vi "L1RightToCargo8.vi"(9 "Initialized":bool) -> (2 "Drive State":T1)   [LabVIEW 2018]
uses:
  driveStateEnum.ctl
  L1RightToCargo8.ctl
  driveShifterEnum.ctl
  HatchPanel/hatchPanelEnum.ctl
  HatchPanel/hatchPanelNotifierCluster.ctl
  MotionProfile/Constants.vi
panel:
  out "Speed (ft/s) 3":dbl=5.820510365604576
  in  "Wait til slower then(ft/s) 3":dbl=-3.0
  out "Speed (ft/s) 2":dbl=5.820510365604576
  in  "Wait til slower then(ft/s) 2":dbl=-3.0
  out "Speed (ft/s)":dbl=5.820510365604576
  in  "Wait til slower then(ft/s)":dbl=-3.0
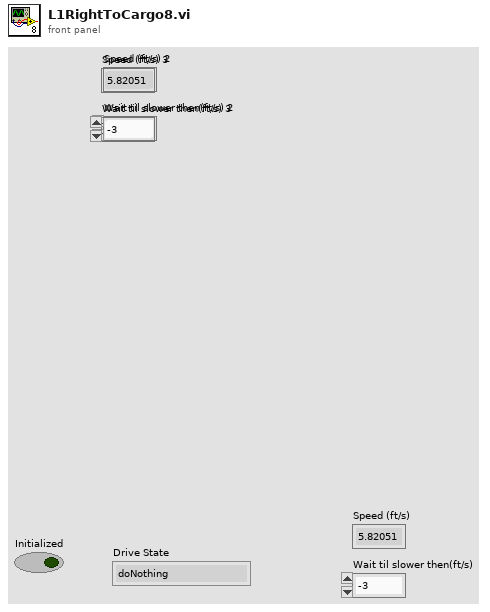
[diagram p1: front panel]
types:
  T1 = typedef "driveStateEnum.ctl" = enum16{"doNothing", "Manuel", "Teleop", "Follow Path (init)", "Follow Path", "Move to Target", "Climb", "Line Align", "Rotate180", "Align50Degrees", "Sonar Brake Tele", "LLCushion", "Auto Approach Target"}
  T2 = typedef "L1RightToCargo8.ctl" = enum16{"7b -  back away from cargo ship ", "1 - MP move to cargo Ship (init)", "2 - MP move to cargo ship", "3 - Delay for shift", "4 - Approach To Score", "5 - Scored", "99 - doNothing", "7a - back away from cargo ship (init)", "8 - Hatch Panel Motion Off", "9 - Scoring Claw On", "8 - turn towards loading station", "10 - Scoring Claw Off", "11 - MP move towards loading station (init)", "12 -  MP move towards loading station", "13 - MP Move towards  cargo ship *2 (init)", "14 - MP Move towards  cargo ship *2"}
  T3 = typedef "WPI_MotorControlDeviceRef.ctl" = cluster{"DeviceStatus":errorcluster, "Type":T4, "PWM":cluster{"PWM Channel":T5, "DeadBand":T6}, "CAN":cluster{"Device Number":u8, "SetOutput VI Ref":variant, "GetOutput VI Ref":variant, "Enable VI Ref":variant, "Disable VI Ref":variant, "Data":variant}, "Invert":bool, "DIO PWM":cluster{"PWM \"Enable\" Channel":T5, "DIOChannel":T7, "PWM Rate":dbl}}
  T4 = typedef "WPI_MotorControlType.ctl" = enum16{"PWM", "CAN", "DIO PWM"}
  T5 = typedef "FPGA_DIOPWMChannel.ctl" = enum8{"PWM 0", "PWM 1", "PWM 2", "PWM 3", "PWM 4", "PWM 5", "PWM 6", "PWM 7", "PWM 8", "PWM 9", "PWM MXP 0", "PWM MXP 1", "PWM MXP 2", "PWM MXP 3", "PWM MXP 4", "PWM MXP 5", "PWM MXP 6", "PWM MXP 7", "PWM MXP 8", "PWM MXP 9", "Invalid"}
  T6 = typedef "WPI_PWMDeadband.ctl" = cluster{"Name":string, "maxPositivePwm":i32, "minPositivePwm":i32, "centerPwm":i32, "maxNegativePwm":i32, "minNegativePwm":i32, "angularRange":u16}
  T7 = typedef "FPGA_DIOChannel.ctl" = enum8{"DIO 0", "DIO 1", "DIO 2", "DIO 3", "DIO 4", "DIO 5", "DIO 6", "DIO 7", "DIO 8", "DIO 9", "DIO MXP 0", "DIO MXP 1", "DIO MXP 2", "DIO MXP 3", "DIO MXP 4", "DIO MXP 5", "DIO MXP 6", "DIO MXP 7", "DIO MXP 8", "DIO MXP 9", "DIO MXP 10", "DIO MXP 11", "DIO MXP 12", "DIO MXP 13", "DIO MXP 14", "DIO MXP 15", "SPI Port CS1", "SPI Port CS2", "SPI Port CS3", "SPI Port MISO", "SPI Port MOSI", "Invalid"}
  T8 = typedef "driveShifterEnum.ctl" = enum16{"Low", "High"}
  T9 = typedef "hatchPanelNotifierCluster.ctl" = cluster{"Hatch Panel State":T10, "Mechanism Motion":bool, "Gathering Claw Motion":bool, "Scoring Claw Motion":bool}
  T10 = typedef "hatchPanelEnum.ctl" = enum16{"do nothing", "State Machine", "Stach Mode", "Climb Mode", "Retracted Closed", "Retracted Open", "Extended Closed", "Extended Open"}
  T11 = typedef "CTRE_PigeonIMU_DeviceRef.ctl" = cluster{"DeviceStatus":errorcluster, "Device Number":u8, "Type":T12, "Device ID":u32, "Handle":u64, "UsageFrame":u32, "Library Path":path}
  T12 = typedef "CTRE_PigeonIMU_ConnectionType.ctl" = u32
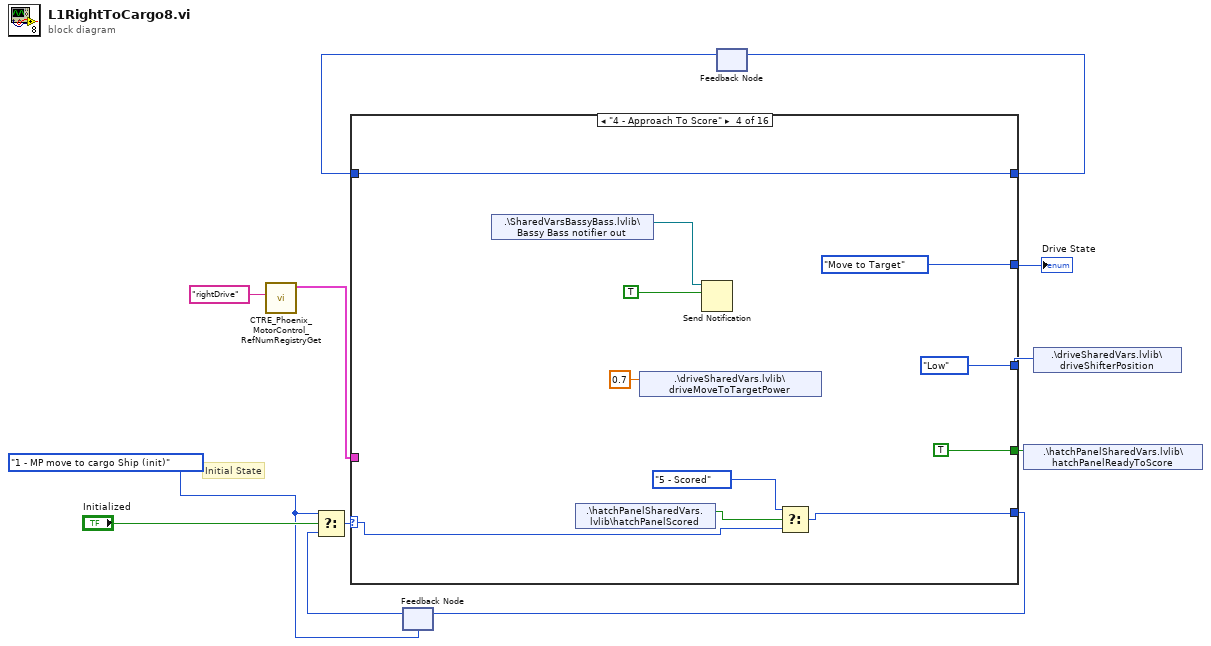
[diagram p0: block diagram]
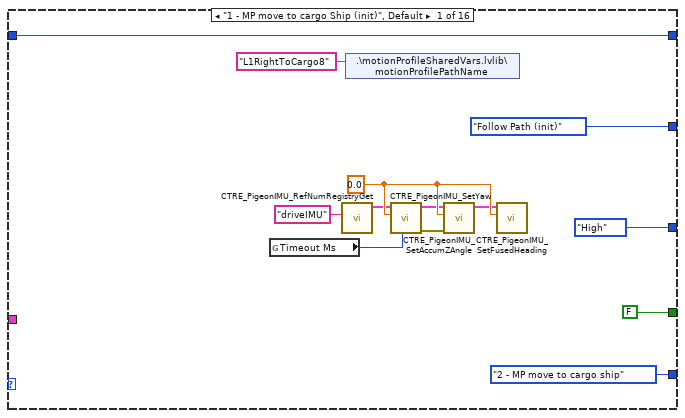
[diagram p2: hidden frame]
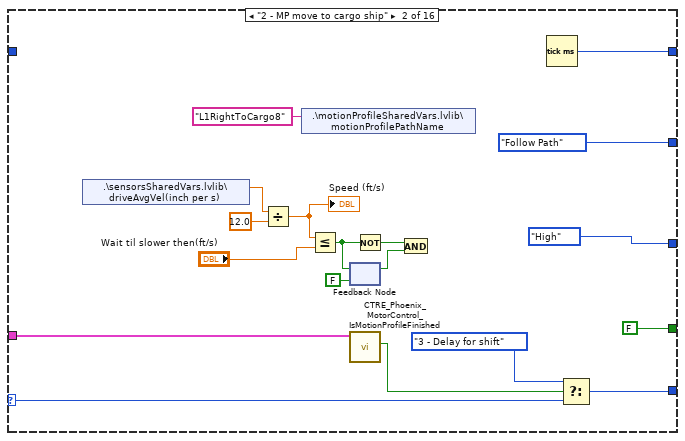
[diagram p3: hidden frame]
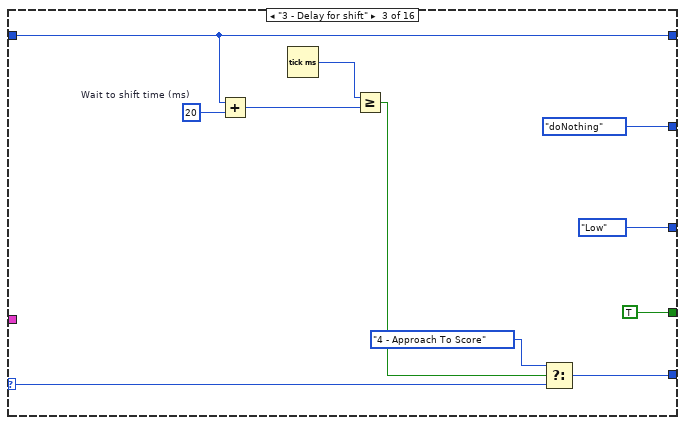
[diagram p4: hidden frame]
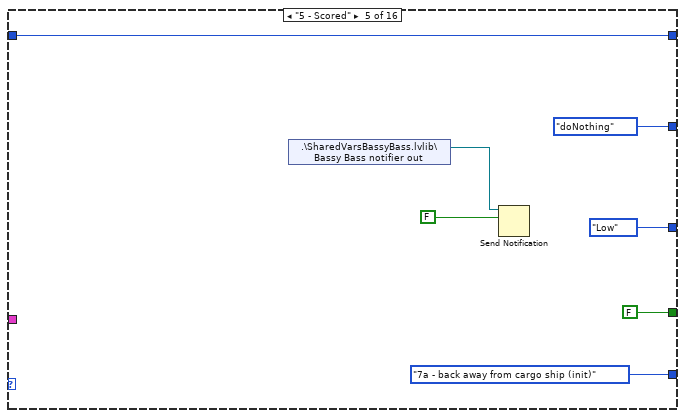
[diagram p5: hidden frame]
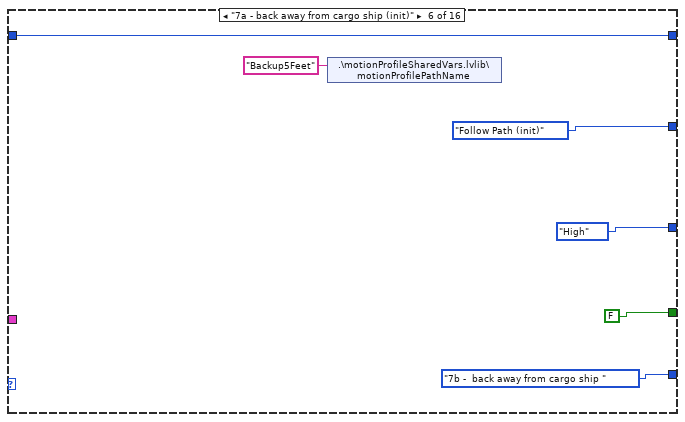
[diagram p6: hidden frame]
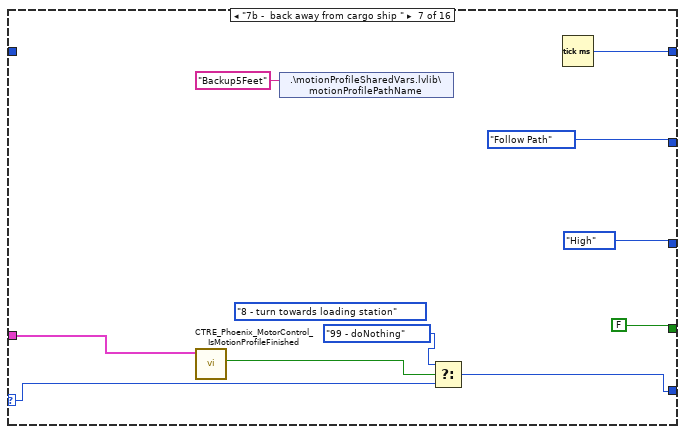
[diagram p7: hidden frame]
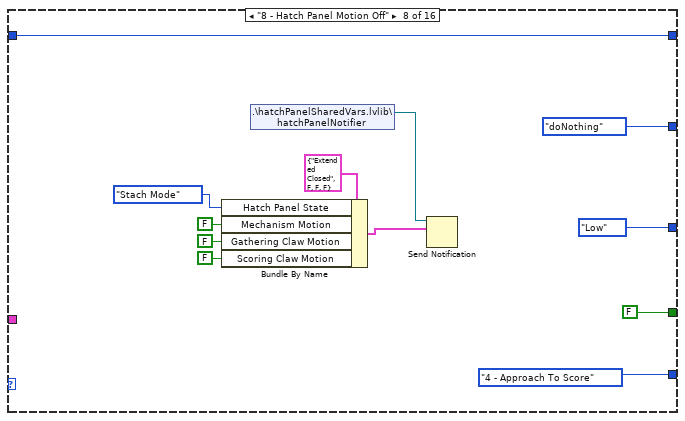
[diagram p8: hidden frame]
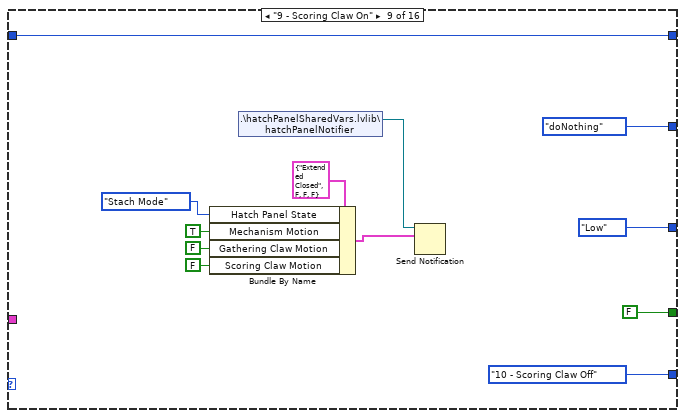
[diagram p9: hidden frame]
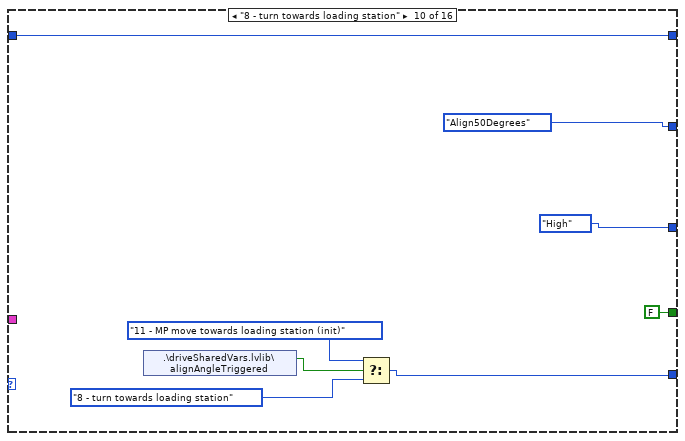
[diagram p10: hidden frame]
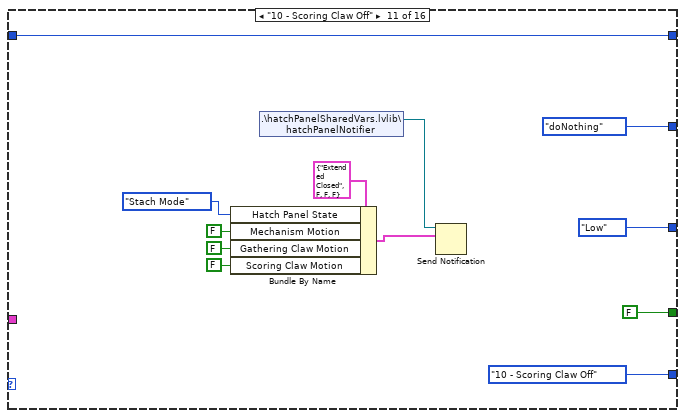
[diagram p11: hidden frame]
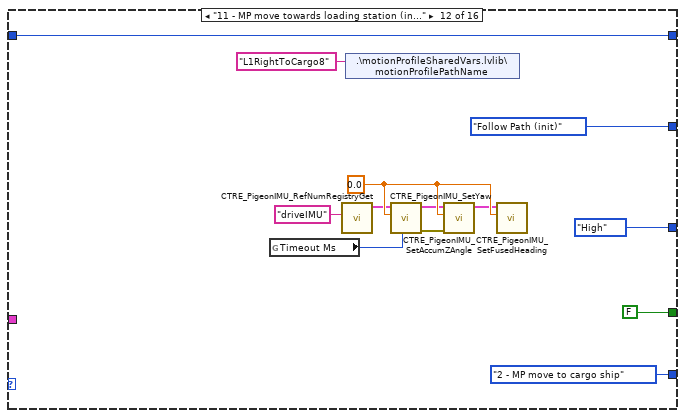
[diagram p12: hidden frame]
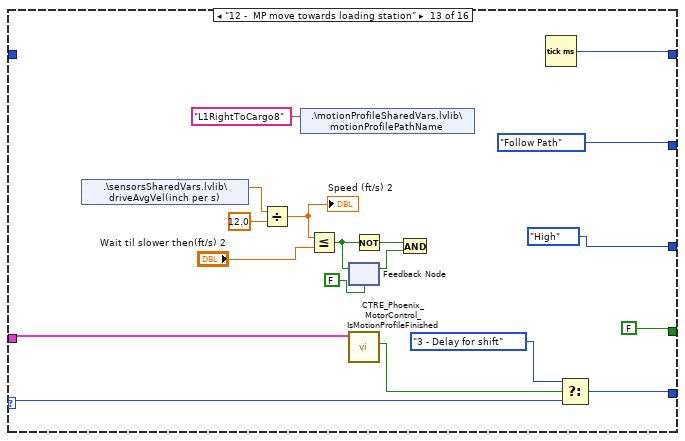
[diagram p13: hidden frame]
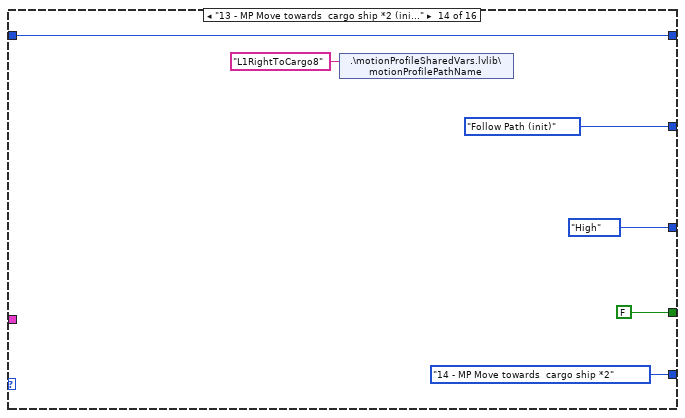
[diagram p14: hidden frame]
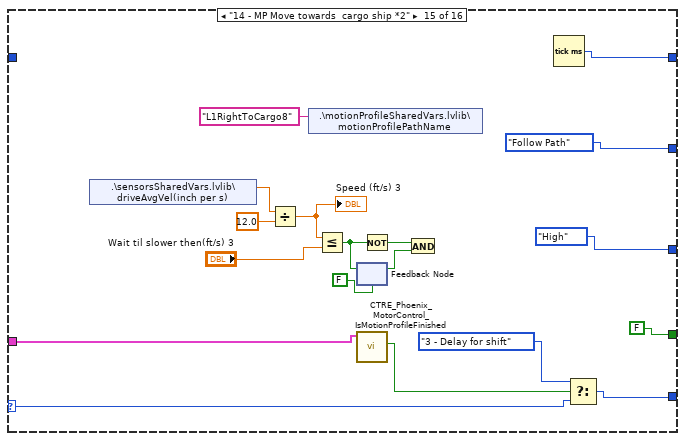
[diagram p15: hidden frame]
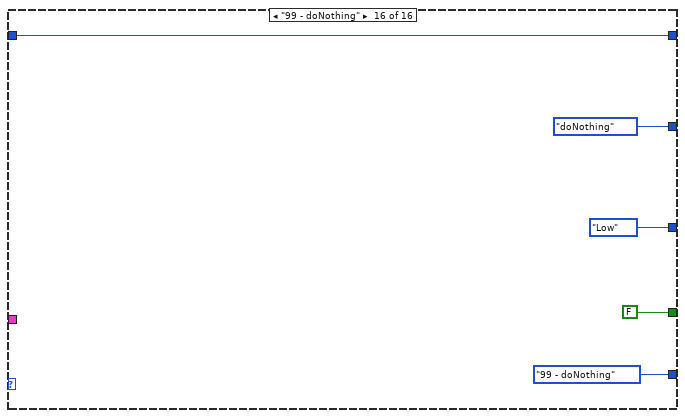
[diagram p16: hidden frame]
diagram:
  w5 = L1RightToCargo8."1 - MP move to cargo Ship (init)" ("Enum")
  # "Initial State"
  n1 = call <vilib>:"CTRE_Phoenix_MotorControl_RefNumRegistryGet.vi"("refnum name"="rightDrive") -> ("PhoenixMotorControlDevRef"=w8:T3)  [unwired: 9 in, 1 out]
  n2 = feedback #1(w5) -> (w11:T2)
  n3 = Select(t=w5, s="Initialized", f=w11) -> (s? t:f=w12:T2)
  n4 = feedback #2() -> (w2:u32)  [unwired: 1 in]
  n5 = case shown="\"4 - Approach To Score\"" w12 {
    selector: w12 -> [_ w41 w46 w59 _ _ w81 _ _ _ _ _ w151 _ w176 _]
    tunnel: [L1RightToCargo8."2 - MP move to cargo ship" ("Enum") w42 w48 w57 L1RightToCargo8."7a - back away from cargo ship (init)" ("Enum") L1RightToCargo8."7b -  back away from cargo ship " ("Enum") w80 L1RightToCargo8."4 - Approach To Score" ("Enum") L1RightToCargo8."10 - Scoring Claw Off" ("Enum") w113 L1RightToCargo8."10 - Scoring Claw Off" ("Enum") L1RightToCargo8."2 - MP move to cargo ship" ("Enum") w152 L1RightToCargo8."14 - MP Move towards  cargo ship *2" ("Enum") w175 L1RightToCargo8."99 - doNothing" ("Enum")] -> w10
    tunnel: [driveStateEnum."Follow Path (init)" ("Drive State Enum") driveStateEnum."Follow Path" ("Drive State Enum") driveStateEnum."doNothing" ("Drive State Enum") driveStateEnum."Move to Target" ("Drive State Enum") driveStateEnum."doNothing" ("Drive State Enum") driveStateEnum."Follow Path (init)" ("Drive State Enum") driveStateEnum."Follow Path" ("Drive State Enum") driveStateEnum."doNothing" ("Drive State Enum") driveStateEnum."doNothing" ("Drive State Enum") driveStateEnum."Align50Degrees" ("Drive State Enum") driveStateEnum."doNothing" ("Drive State Enum") driveStateEnum."Follow Path (init)" ("Drive State Enum") driveStateEnum."Follow Path" ("Drive State Enum") driveStateEnum."Follow Path (init)" ("Drive State Enum") driveStateEnum."Follow Path" ("Drive State Enum") driveStateEnum."doNothing" ("Drive State Enum")] -> w6
    tunnel: w8 -> [_ w39 _ _ _ _ w82 _ _ _ _ _ w150 _ w170 _]
    tunnel: [driveShifterEnum."High" ("driveShifterPosition") driveShifterEnum."High" ("driveShifterPosition") driveShifterEnum."Low" ("driveShifterPosition") driveShifterEnum."Low" ("driveShifterPosition") driveShifterEnum."Low" ("driveShifterPosition") driveShifterEnum."High" ("driveShifterPosition") driveShifterEnum."High" ("driveShifterPosition") driveShifterEnum."Low" ("driveShifterPosition") driveShifterEnum."Low" ("driveShifterPosition") driveShifterEnum."High" ("driveShifterPosition") driveShifterEnum."Low" ("driveShifterPosition") driveShifterEnum."High" ("driveShifterPosition") driveShifterEnum."High" ("driveShifterPosition") driveShifterEnum."High" ("driveShifterPosition") driveShifterEnum."High" ("driveShifterPosition") driveShifterEnum."Low" ("driveShifterPosition")] -> w4
    tunnel: [w14 w27 w52 w63 w68 w77 w83 w93 w105 w119 w122 w134 w147 w168 w171 w188] -> w3
    tunnel: w2 -> [w14 _ w52 w63 w68 w77 _ w93 w105 w119 w122 w134 _ w168 _ w188]
    tunnel: [FALSE FALSE TRUE TRUE FALSE FALSE FALSE FALSE FALSE FALSE FALSE FALSE FALSE FALSE FALSE FALSE] -> w1
    frame "1 - MP move to cargo Ship (init)", Default {
      w23 = 0.0 ("Angle (Deg)")
      n6 = global read "Constants.vi" "Timeout Ms"() -> (w20:i32)
      n7 = call <vilib>:"CTRE_PigeonIMU_RefNumRegistryGet.vi"("refnum name"="driveIMU") -> ("PigeonIMUDevRef"=w17:T11)  [unwired: 9 in, 1 out]
      n8 = shared-variable ".\\motionProfileSharedVars.lvlib\\motionProfilePathName"("L1RightToCargo8" ("motionProfilePathName")) -> ()  [unwired: 1 in, 1 out]
      n9 = call <vilib>:"CTRE_PigeonIMU_SetYaw.vi"("timeoutMs"=w20, "Value"=w23, "PigeonIMUDevRef"=w17) -> ("error out"=w18:errorcluster, "PigeonIMUDevRef"=w19:T11)  [unwired: 7 in]
      n10 = call <vilib>:"CTRE_PigeonIMU_SetAccumZAngle.vi"("error in (no error)"=w18, "Angle (Deg)"=w23, "PigeonIMUDevRef"=w19) -> ("PigeonIMUDevRef"=w21:T11)  [unwired: 7 in, 1 out]
      n11 = call <vilib>:"CTRE_PigeonIMU_SetFusedHeading.vi"("Value"=w23, "PigeonIMUDevRef 2"=w21) -> ()  [unwired: 8 in, 2 out]
    }
    frame "2 - MP move to cargo ship" {
      n12 = shared-variable ".\\sensorsSharedVars.lvlib\\driveAvgVel(inch per s)"() -> (w38:dbl)  [unwired: 1 in, 1 out]
      n13 = Divide(x=w38, y=12.0) -> (x/y=w36:dbl)
      "Speed (ft/s)" <- w36
      n14 = shared-variable ".\\motionProfileSharedVars.lvlib\\motionProfilePathName"("L1RightToCargo8" ("motionProfilePathName")) -> ()  [unwired: 1 in, 1 out]
      n15 = Less Or Equal?(x=w36, y="Wait til slower then(ft/s)") -> (x <= y?=w33:bool)
      n16 = feedback-in #3(w33) -> ()
      n17 = feedback #3(FALSE) -> (w32:bool)
      n18 = call <vilib>:"CTRE_Phoenix_MotorControl_IsMotionProfileFinished.vi"("PhoenixMotorControlDevRef"=w39) -> ("Is Motion Profile Finished?"=w30:bool)  [unwired: 8 in, 2 out]
      n19 = Not(x=w33) -> (.not. x?=w31:bool)
      n20 = And(x=w31, y=w32) -> ()  [unwired: 1 out]
      n21 = Tick Count (ms)() -> (millisecond timer value=w27:u32)
      n22 = Select(t=L1RightToCargo8."3 - Delay for shift", s=w30, f=w41) -> (s? t:f=w42:T2)
    }
    frame "3 - Delay for shift" {
      w51 = u32 20  # Wait to shift time (ms)
      n23 = Add(x=w52, y=w51) -> (x+y=w49:u32)
      n24 = Tick Count (ms)() -> (millisecond timer value=w50:u32)
      n25 = Greater Or Equal?(x=w50, y=w49) -> (x >= y?=w47:bool)
      n26 = Select(t=L1RightToCargo8."4 - Approach To Score", s=w47, f=w46) -> (s? t:f=w48:T2)
    }
    frame "4 - Approach To Score" {
      n27 = shared-variable ".\\SharedVarsBassyBass.lvlib\\Bassy Bass notifier out"() -> (w56:refnum<notifier>)  [unwired: 1 in, 1 out]
      n28 = shared-variable ".\\hatchPanelSharedVars.lvlib\\hatchPanelScored"() -> (w60:bool)  [unwired: 1 in, 1 out]
      n29 = shared-variable ".\\driveSharedVars.lvlib\\driveMoveToTargetPower"(0.7 ("driveMoveToTargetPower")) -> ()  [unwired: 1 in, 1 out]
      n30 = Send Notification(notification=TRUE, notifier=w56) -> ()  [unwired: 1 in, 2 out]
      n31 = Select(t=L1RightToCargo8."5 - Scored" ("Enum"), s=w60, f=w59) -> (s? t:f=w57:T2)
    }
    frame "5 - Scored" {
      n32 = shared-variable ".\\SharedVarsBassyBass.lvlib\\Bassy Bass notifier out"() -> (w67:refnum<notifier>)  [unwired: 1 in, 1 out]
      n33 = Send Notification(notification=FALSE, notifier=w67) -> ()  [unwired: 1 in, 2 out]
    }
    frame "7a - back away from cargo ship (init)" {
      n34 = shared-variable ".\\motionProfileSharedVars.lvlib\\motionProfilePathName"("Backup5Feet" ("motionProfilePathName")) -> ()  [unwired: 1 in, 1 out]
    }
    frame "7b -  back away from cargo ship " {
      (unwired) L1RightToCargo8."8 - turn towards loading station" ("t")
      n35 = call <vilib>:"CTRE_Phoenix_MotorControl_IsMotionProfileFinished.vi"("PhoenixMotorControlDevRef"=w82) -> ("Is Motion Profile Finished?"=w85:bool)  [unwired: 8 in, 2 out]
      n36 = shared-variable ".\\motionProfileSharedVars.lvlib\\motionProfilePathName"("Backup5Feet" ("motionProfilePathName")) -> ()  [unwired: 1 in, 1 out]
      n37 = Select(t=L1RightToCargo8."99 - doNothing", s=w85, f=w81) -> (s? t:f=w80:T2)
      n38 = Tick Count (ms)() -> (millisecond timer value=w83:u32)
    }
    frame "8 - Hatch Panel Motion Off" {
      n39 = Bundle By Name(cluster=T9 {"Hatch Panel State"=enum."Extended Closed", "Mechanism Motion"=FALSE, "Gathering Claw Motion"=FALSE, "Scoring Claw Motion"=FALSE} ("notification"), "Hatch Panel State"=hatchPanelEnum."Stach Mode", "Mechanism Motion"=FALSE, "Gathering Claw Motion"=FALSE, "Scoring Claw Motion"=FALSE) -> (w97:T9)
      n40 = shared-variable ".\\hatchPanelSharedVars.lvlib\\hatchPanelNotifier"() -> (w98:refnum<notifier>)  [unwired: 1 in, 1 out]
      n41 = Send Notification(notification=w97, notifier=w98) -> ()  [unwired: 1 in, 2 out]
    }
    frame "9 - Scoring Claw On" {
      n42 = Bundle By Name(cluster=T9 {"Hatch Panel State"=enum."Extended Closed", "Mechanism Motion"=FALSE, "Gathering Claw Motion"=FALSE, "Scoring Claw Motion"=FALSE} ("notification"), "Hatch Panel State"=hatchPanelEnum."Stach Mode", "Mechanism Motion"=TRUE, "Gathering Claw Motion"=FALSE, "Scoring Claw Motion"=FALSE) -> (w109:T9)
      n43 = shared-variable ".\\hatchPanelSharedVars.lvlib\\hatchPanelNotifier"() -> (w110:refnum<notifier>)  [unwired: 1 in, 1 out]
      n44 = Send Notification(notification=w109, notifier=w110) -> ()  [unwired: 1 in, 2 out]
    }
    frame "8 - turn towards loading station" {
      n45 = shared-variable ".\\driveSharedVars.lvlib\\alignAngleTriggered"() -> (w116:bool)  [unwired: 1 in, 1 out]
      n46 = Select(t=L1RightToCargo8."11 - MP move towards loading station (init)" ("Enum"), s=w116, f=L1RightToCargo8."8 - turn towards loading station" ("Enum")) -> (s? t:f=w113:T2)
    }
    frame "10 - Scoring Claw Off" {
      n47 = Bundle By Name(cluster=T9 {"Hatch Panel State"=enum."Extended Closed", "Mechanism Motion"=FALSE, "Gathering Claw Motion"=FALSE, "Scoring Claw Motion"=FALSE} ("notification"), "Hatch Panel State"=hatchPanelEnum."Stach Mode", "Mechanism Motion"=FALSE, "Gathering Claw Motion"=FALSE, "Scoring Claw Motion"=FALSE) -> (w129:T9)
      n48 = shared-variable ".\\hatchPanelSharedVars.lvlib\\hatchPanelNotifier"() -> (w130:refnum<notifier>)  [unwired: 1 in, 1 out]
      n49 = Send Notification(notification=w129, notifier=w130) -> ()  [unwired: 1 in, 2 out]
    }
    frame "11 - MP move towards loading station (init)" {
      w143 = 0.0 ("Angle (Deg)")
      n50 = global read "Constants.vi" "Timeout Ms"() -> (w140:i32)
      n51 = call <vilib>:"CTRE_PigeonIMU_RefNumRegistryGet.vi"("refnum name"="driveIMU") -> ("PigeonIMUDevRef"=w137:T11)  [unwired: 9 in, 1 out]
      n52 = shared-variable ".\\motionProfileSharedVars.lvlib\\motionProfilePathName"("L1RightToCargo8" ("motionProfilePathName")) -> ()  [unwired: 1 in, 1 out]
      n53 = call <vilib>:"CTRE_PigeonIMU_SetYaw.vi"("timeoutMs"=w140, "Value"=w143, "PigeonIMUDevRef"=w137) -> ("error out"=w138:errorcluster, "PigeonIMUDevRef"=w139:T11)  [unwired: 7 in]
      n54 = call <vilib>:"CTRE_PigeonIMU_SetAccumZAngle.vi"("error in (no error)"=w138, "Angle (Deg)"=w143, "PigeonIMUDevRef"=w139) -> ("PigeonIMUDevRef"=w141:T11)  [unwired: 7 in, 1 out]
      n55 = call <vilib>:"CTRE_PigeonIMU_SetFusedHeading.vi"("Value"=w143, "PigeonIMUDevRef 2"=w141) -> ()  [unwired: 8 in, 2 out]
    }
    frame "12 -  MP move towards loading station" {
      n56 = shared-variable ".\\sensorsSharedVars.lvlib\\driveAvgVel(inch per s)"() -> (w157:dbl)  [unwired: 1 in, 1 out]
      n57 = Divide(x=w157, y=12.0) -> (x/y=w158:dbl)
      "Speed (ft/s) 2" <- w158
      n58 = shared-variable ".\\motionProfileSharedVars.lvlib\\motionProfilePathName"("L1RightToCargo8" ("motionProfilePathName")) -> ()  [unwired: 1 in, 1 out]
      n59 = Less Or Equal?(x=w158, y="Wait til slower then(ft/s) 2") -> (x <= y?=w160:bool)
      n60 = feedback #4(FALSE) -> (w161:bool)
      n61 = feedback-in #4(w160) -> ()
      n62 = call <vilib>:"CTRE_Phoenix_MotorControl_IsMotionProfileFinished.vi"("PhoenixMotorControlDevRef"=w150) -> ("Is Motion Profile Finished?"=w163:bool)  [unwired: 8 in, 2 out]
      n63 = Not(x=w160) -> (.not. x?=w162:bool)
      n64 = And(x=w162, y=w161) -> ()  [unwired: 1 out]
      n65 = Tick Count (ms)() -> (millisecond timer value=w147:u32)
      n66 = Select(t=L1RightToCargo8."3 - Delay for shift", s=w163, f=w151) -> (s? t:f=w152:T2)
    }
    frame "13 - MP Move towards  cargo ship *2 (init)" {
      n67 = shared-variable ".\\motionProfileSharedVars.lvlib\\motionProfilePathName"("L1RightToCargo8" ("motionProfilePathName")) -> ()  [unwired: 1 in, 1 out]
    }
    frame "14 - MP Move towards  cargo ship *2" {
      n68 = shared-variable ".\\sensorsSharedVars.lvlib\\driveAvgVel(inch per s)"() -> (w181:dbl)  [unwired: 1 in, 1 out]
      n69 = Divide(x=w181, y=12.0) -> (x/y=w182:dbl)
      "Speed (ft/s) 3" <- w182
      n70 = shared-variable ".\\motionProfileSharedVars.lvlib\\motionProfilePathName"("L1RightToCargo8" ("motionProfilePathName")) -> ()  [unwired: 1 in, 1 out]
      n71 = Less Or Equal?(x=w182, y="Wait til slower then(ft/s) 3") -> (x <= y?=w184:bool)
      n72 = feedback #5(FALSE) -> (w185:bool)
      n73 = feedback-in #5(w184) -> ()
      n74 = call <vilib>:"CTRE_Phoenix_MotorControl_IsMotionProfileFinished.vi"("PhoenixMotorControlDevRef"=w170) -> ("Is Motion Profile Finished?"=w187:bool)  [unwired: 8 in, 2 out]
      n75 = Not(x=w184) -> (.not. x?=w186:bool)
      n76 = And(x=w186, y=w185) -> ()  [unwired: 1 out]
      n77 = Tick Count (ms)() -> (millisecond timer value=w171:u32)
      n78 = Select(t=L1RightToCargo8."3 - Delay for shift", s=w187, f=w176) -> (s? t:f=w175:T2)
    }
    frame "99 - doNothing" {
    }
  }
  "Drive State" <- w6
  n79 = feedback-in #1(w10) -> ()
  n80 = feedback-in #2(w3) -> ()
  n81 = shared-variable ".\\hatchPanelSharedVars.lvlib\\hatchPanelReadyToScore"(w1) -> ()  [unwired: 1 in, 1 out]
  n82 = shared-variable ".\\driveSharedVars.lvlib\\driveShifterPosition"(w4) -> ()  [unwired: 1 in, 1 out]
